vi "Format Log XY Data.vi"(6 "Sweeping?":bool, 8 "error in (no error)":errorcluster, 9 "Y":waveform(dbl)[](array[waveform]), 10 "X":waveform(dbl)[](array[waveform]), 11 "Instrument.Lockin in":refnum<class "Instrument.Lockin.lvclass">) -> (0 "error out":errorcluster, 1 "Log Data":T1[](array[typedef]), 2 "Log Paths":string, 3 "Instrument.Lockin out":refnum<class "Instrument.Lockin.lvclass">, 4 "Times":timestamp[](array[timestamp]) format="%<%.6X\n%x>T")   [LabVIEW 2019, in "Instrument.Lockin.lvlib" / "Instrument.Lockin.lvclass"]
uses:
  Instrument.Lockin.lvclass
  Typedefs/Lockin.LogSweepXY--Cluster.ctl
  Instrument.Lockin.lvclass/Instrument.Lockin.ctl
  Generator/Generator.lvclass
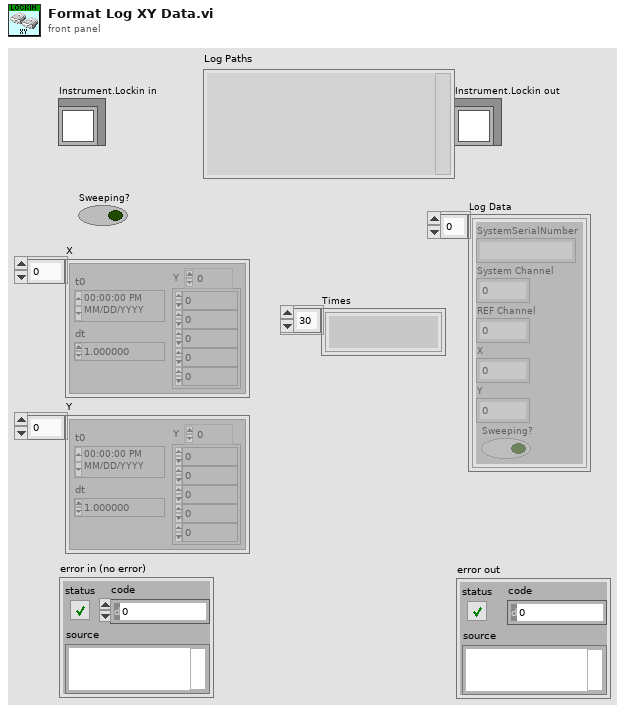
[diagram p1: front panel]
types:
  T1 = typedef "Instrument.Lockin.lvlib/Instrument.Lockin.lvclass/Lockin.LogSweepXY--Cluster.ctl" = cluster{"SystemSerialNumber":string, "System Channel":i32, "REF Channel":i32, "X":dbl, "Y":dbl, "Sweeping?":bool}
  T2 = typedef "Instrument.Lockin.lvlib/Instrument.DAQ.lvclass/DeviceInfo--Cluster.ctl" = cluster{"DeviceName":string, "DevIsSimulated":bool, "DeviceSerialNumber":string, "ProductType":string, "ProductCategory":i32, "ProductNumber":u32, "ChassisNumber":u32, "SlotNumber":u32, "ChassisName":string, "ChassisSerialNumber":string, "DevTemp":dbl, "SelfCal.LastDate/Time":string, "SelfCal.LastTemp":dbl, "calibration due?":bool}
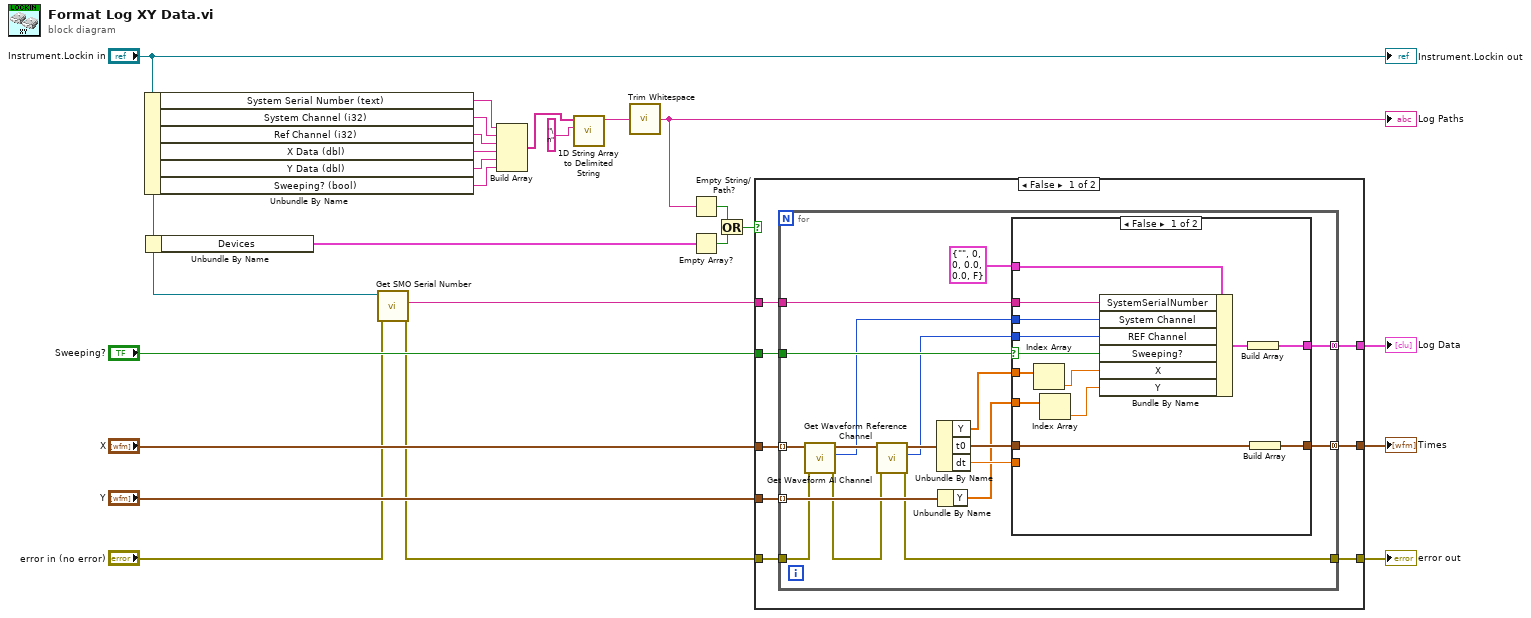
[diagram p0: block diagram]
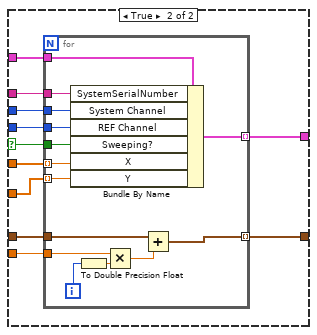
[diagram p2: hidden frame]
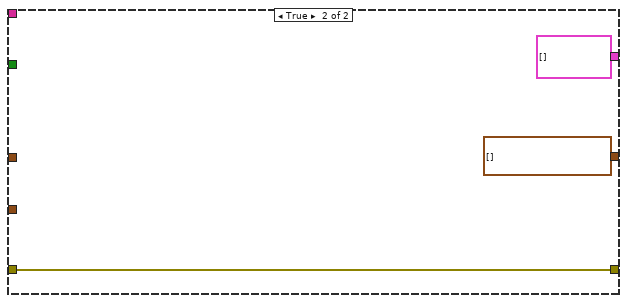
[diagram p3: hidden frame]
diagram:
  n1 = Unbundle By Name("Instrument.Lockin in") -> ("System Serial Number (text)"=w18:string, "System Channel (i32)"=w5:string, "Ref Channel (i32)"=w4:string, "X Data (dbl)"=w3:string, "Y Data (dbl)"=w2:string, "Sweeping? (bool)"=w1:string)
  n2 = Unbundle By Name("Instrument.Lockin in") -> ("Devices"=w12:T2[])
  n3 = call-dynamic "Get SMO Serial Number.vi"("error in (no error)"="error in (no error)", "Instrument.Lockin in"="Instrument.Lockin in") -> ("error out"=w6:errorcluster, "Serial Number"=w8:string)  [unwired: 7 in, 1 out]
  n4 = Build Array(w18, w5, w4, w3, w2, w1) -> (w17:string[])
  n5 = call <vilib>:"1D String Array to Delimited String.vi"("delimiter"="\n", "string array"=w17) -> ("delimited string"=w11:string)  [unwired: 9 in]
  n6 = call <vilib>:"Trim Whitespace.vi"("string"=w11) -> ("trimmed string"=w10:string)  [unwired: 1 in]
  "Log Paths" <- w10
  n7 = Empty String/Path?(string/path=w10) -> (empty?=w14:bool)
  n8 = Empty Array?(array=w12) -> (empty?=w15:bool)
  n9 = Or(x=w14, y=w15) -> (x .or. y?=w13:bool)
  n10 = case shown="False" w13 {
    tunnel: [w32 timestamp[] []] -> w24
    tunnel: "Sweeping?" -> [w31 _]
    tunnel: [w30 T1[] []] -> w22
    tunnel: w8 -> [w29 _]
    tunnel: "Y" -> [w28 _]
    tunnel: "X" -> [w27 _]
    tunnel: w6 -> [w26 w90]
    tunnel: [w25 w90] -> w19
    frame False {
      n11 = for {
        tunnel: [w50] -> w32 mode=concatenating
        tunnel: w31 -> [w49]
        tunnel: [w48] -> w30 mode=concatenating
        tunnel: w29 -> [w47]
        tunnel: w28 -> [w46] mode=indexing
        tunnel: w27 -> [w39] mode=indexing
        tunnel: w26 -> [w36]
        tunnel: [w34] -> w25
        n12 = call "Get Waveform AI Channel.vi"("error in (no error)"=w36, "Reference in"=w39) -> ("error out"=w35:errorcluster, "AI Channel"=w37:i32, "Reference out"=w41:waveform(dbl))  [unwired: 7 in]
        n13 = call "Get Waveform Reference Channel.vi"("error in (no error)"=w35, "Reference in"=w41) -> ("error out"=w34:errorcluster, "Reference Channel"=w38:i32, "Reference out"=w40:waveform(dbl))  [unwired: 7 in]
        n14 = Unbundle By Name(w40) -> ("Y"=w42:dbl[], "t0"=w45:timestamp, "dt"=w44:dbl)
        n15 = Unbundle By Name(w46) -> ("Y"=w43:dbl[])
        n16 = case shown="False" w49 {
          selector: w49 -> [w57 w73]
          tunnel: [w56 w74] -> w50
          tunnel: w37 -> [w59 w72]
          tunnel: w44 -> [_ w71]
          tunnel: w45 -> [w55 w70]
          tunnel: [w62 w69] -> w48
          tunnel: w43 -> [w52 w68]
          tunnel: w38 -> [w58 w67]
          tunnel: T1 {"SystemSerialNumber"="", "System Channel"=0, "REF Channel"=0, "X"=0.0, "Y"=0.0, "Sweeping?"=FALSE} ("cluster") -> [w63 w66]
          tunnel: w42 -> [w54 w65]
          tunnel: w47 -> [w60 w64]
          frame False {
            n17 = Index Array(array=w54) -> (element=w53:dbl)  [unwired: 1 in]
            n18 = Index Array(array=w52) -> (element=w51:dbl)  [unwired: 1 in]
            n19 = Bundle By Name(cluster=w63, "SystemSerialNumber"=w60, "System Channel"=w59, "REF Channel"=w58, "Sweeping?"=w57, "X"=w53, "Y"=w51) -> (w61:T1)
            n20 = Build Array(w61) -> (w62:T1[])
            n21 = Build Array(w55) -> (w56:timestamp[])
          }
          frame True {
            n22 = for {
              tunnel: w70 -> [w84]
              tunnel: w71 -> [w88]
              tunnel: [w75] -> w74 mode=indexing
              tunnel: w65 -> [w81] mode=indexing
              tunnel: w64 -> [w78]
              tunnel: w72 -> [w79]
              tunnel: w73 -> [w83]
              tunnel: [w82] -> w69 mode=indexing
              tunnel: w68 -> [w80] mode=indexing
              tunnel: w67 -> [w77]
              tunnel: w66 -> [w76]
              i -> [w87]
              n23 = Bundle By Name(cluster=w76, "SystemSerialNumber"=w78, "System Channel"=w79, "REF Channel"=w77, "Sweeping?"=w83, "X"=w81, "Y"=w80) -> (w82:T1)
              n24 = To Double Precision Float(number=w87) -> (double precision float=w86:dbl)
              n25 = Multiply(x=w88, y=w86) -> (x*y=w85:dbl)
              n26 = Add(x=w84, y=w85) -> (x+y=w75:timestamp)
            }
          }
        }
      }
    }
    frame True {
    }
  }
  "Times" <- w24
  "Log Data" <- w22
  "error out" <- w19
  "Instrument.Lockin out" <- "Instrument.Lockin in"
